vi "Transfer Viewable Resources.vi"(10 "Recipient Viewable In":refnum<class "IViewable.lvclass">, 11 "Running Viewable":refnum<class "IViewable.lvclass">) -> (2 "Recipient Viewable Out":refnum<class "IViewable.lvclass">)   [LabVIEW 2020, in "MVA Framework.lvlib" / "IViewable.lvlib" / "IViewable.lvclass"]
doc: "转移可查看资源"
uses:
  IViewable.lvclass
  IViewable.lvclass/IViewable.ctl
  mva-core/Source/IObserver/IObserver/IObserver.lvclass/IObserver.ctl
  mva-core/Source/IObserver/IObserver/IObserver.lvclass
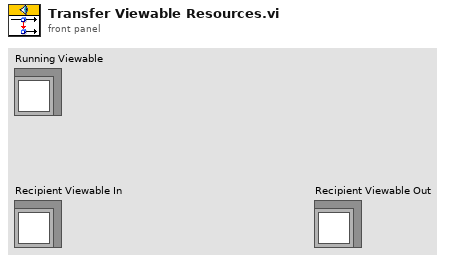
[diagram p1: front panel]
types:
  T1 = typedef "MVA Framework.lvlib/IViewable.lvlib/ApplicationStyleReference.lvclass/Application Style Reference.ctl" = refnum<data-value>
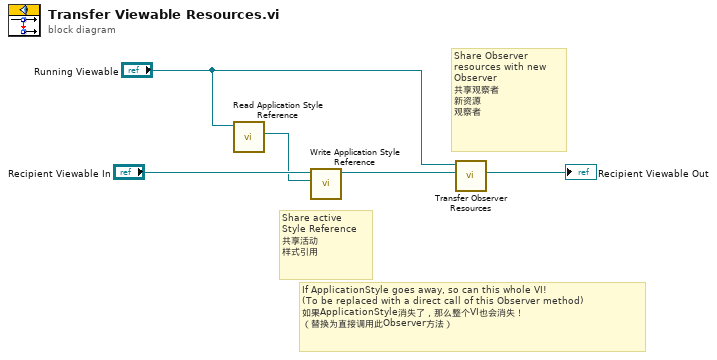
[diagram p0: block diagram]
diagram:
  # "If ApplicationStyle goes away, so can this whole VI!\n(To be replaced with a direct call of this Observer method)\n如果ApplicationStyle消失了，那么整个VI也会消失！\n（替换为直接调用此Observer方法）"
  # "Share Observer\nresources with new\nObserver\n共享观察者\n新资源\n观察者"
  # "Share active\nStyle Reference\n共享活动\n样式引用"
  n1 = call "Read Application Style Reference.vi"("IViewable in"="Running Viewable") -> ("Application Style Reference"=w4:T1)  [unwired: 10 in]
  n2 = call "Write Application Style Reference.vi"("Application Style Reference"=w4, "IViewable in"="Recipient Viewable In") -> ("IViewable out"=w2:refnum<class "IViewable.lvclass">)  [unwired: 9 in]
  n3 = call "Transfer Observer Resources.vi"("Recipient Observer In"=w2, "Running Observer"="Running Viewable") -> ("Recipient Observer Out"=→"Recipient Viewable Out":refnum<class "IViewable.lvclass">)  [unwired: 9 in]
